vi "Read List Information.vi"(8 "Sequence":bool, 9 "Index":i32, 10 "Symbol":string, 11 "Explanation":string) -> (0 "error out":errorcluster, 3 "Program+NO.+Symbol+Explanation":string[](array[string]))   [LabVIEW 2017]
uses:
  <vilib>/Utility/xml.llb/Read From XML File(array).vi
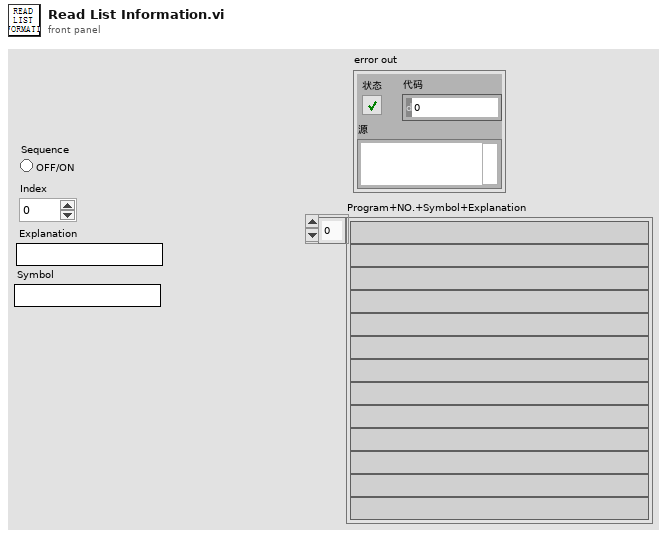
[diagram p1: front panel]
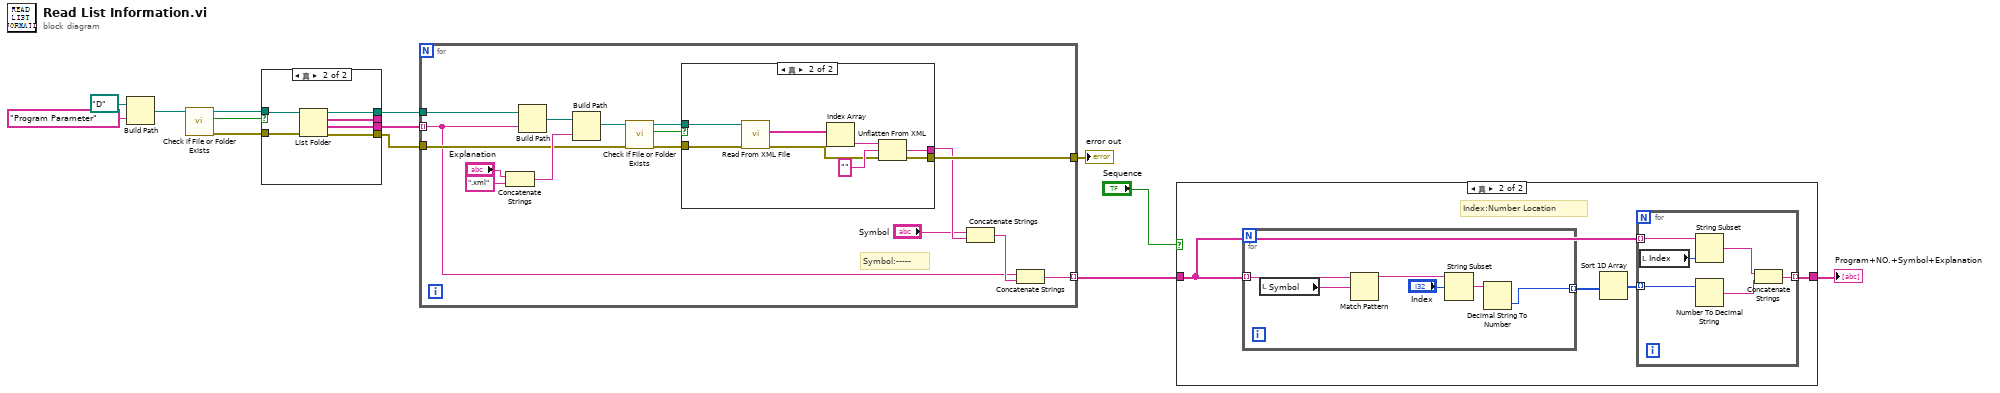
[diagram p0: block diagram]
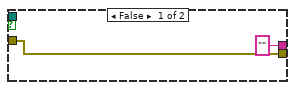
[diagram p3: hidden frame]
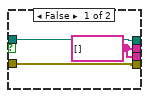
[diagram p4: hidden frame]
diagram:
  n1 = Build Path(base path=path "D:/" ("基路径"), name or relative path="Program Parameter" ("名称或相对路径")) -> (appended path=w11:path)
  n2 = call <vilib>:"Check if File or Folder Exists.vi"("path"=w11) -> ("error out"=w8:errorcluster, "file or folder exists?"=w10:bool, "dup path"=w9:path)  [unwired: 8 in]
  n3 = case shown="真" w10 {
    tunnel: w9 -> [w16 w22]
    tunnel: w8 -> [w15 w21]
    tunnel: [w16 w20] -> w6
    tunnel: [w14 w19] -> _
    tunnel: [w14 w18] -> w7
    tunnel: [w15 w17] -> w5
    frame False {
      w14 = string[] [] ("filenames")
    }
    frame True {
      n4 = List Folder(path=w22, error in=w21) -> (path out=w20:path, filenames=w19:string[], folder names=w18:string[], error out=w17:errorcluster)  [unwired: 2 in]
    }
  }
  n5 = for {
    tunnel: w7 -> [w24] mode=indexing
    tunnel: w6 -> [w38]
    tunnel: w5 -> [w32]
    tunnel: [w28] -> w3
    tunnel: [w23] -> w2 mode=indexing
    # "Symbol:-----"
    n6 = Concatenate Strings("Explanation", ".xml" ("字符串")) -> (w36:string)
    n7 = Build Path(base path=w38, name or relative path=w24) -> (appended path=w37:path)
    n8 = Build Path(base path=w37, name or relative path=w36) -> (appended path=w33:path)
    n9 = call <vilib>:"Check if File or Folder Exists.vi"("error in (no error)"=w32, "path"=w33) -> ("error out"=w29:errorcluster, "file or folder exists?"=w31:bool, "dup path"=w30:path)  [unwired: 7 in]
    n10 = case shown="真" w31 {
      tunnel: w30 -> [_ w48]
      tunnel: w29 -> [w40 w47]
      tunnel: [w40 w42] -> w28
      tunnel: ["" w41] -> w27
      frame False {
      }
      frame True {
        n11 = call-poly <vilib>:"Read From XML File.vi"("error in (no error)"=w47, "XML File Path"=w48) -> ("error out"=w43:errorcluster, "XML Elements"=w46:string[])  [unwired: 7 in, 1 out]
        n12 = Index Array(array=w46) -> (element=w45:string)  [unwired: 1 in]
        n13 = Unflatten From XML(xml string=w45, type="", error in (no error)=w43) -> (value=w41:string, error out=w42:errorcluster)
      }
    }
    n14 = Concatenate Strings("Symbol", w27) -> (w25:string)
    n15 = Concatenate Strings(w24, w25) -> (w23:string)
  }
  "error out" <- w3
  n16 = case shown="真" "Sequence" {
    tunnel: w2 -> [w49 w51]
    tunnel: [w49 w50] -> w1
    frame False {
    }
    frame True {
      # "Index:Number Location"
      n17 = for {
        tunnel: w51 -> [w62] mode=indexing
        tunnel: [w64] -> w52 mode=indexing
        n18 = local read "Symbol"() -> (w61:string)
        n19 = Match Pattern(string=w62, regular expression=w61) -> (before substring=w60:string)  [unwired: 1 in, 3 out]
        n20 = String Subset(string=w60, offset (0)="Index") -> (substring=w65:string)  [unwired: 1 in]
        n21 = Decimal String To Number(string=w65) -> (number=w64:i32)  [unwired: 2 in, 1 out]
      }
      n22 = Sort 1D Array(array=w52) -> (sorted array=w53:i32[])
      n23 = for {
        tunnel: w53 -> [w59] mode=indexing
        tunnel: w51 -> [w58] mode=indexing
        tunnel: [w55] -> w50 mode=indexing
        n24 = local read "Index"() -> (w54:i32)
        n25 = String Subset(string=w58, length (rest)=w54) -> (substring=w57:string)  [unwired: 1 in]
        n26 = Number To Decimal String(number=w59) -> (decimal integer string=w56:string)  [unwired: 1 in]
        n27 = Concatenate Strings(w57, w56) -> (w55:string)
      }
    }
  }
  "Program+NO.+Symbol+Explanation" <- w1
